vi "TestStand.Shutdown.vi"(8 "error in (no error)":errorcluster, 11 "state variables in":T1={"Main.DUTs"=[], "Pages.Name"=[], "Pages.Ref"=[], "TS.UI"={"References"={"Event Callback"=refnum, "Quit Application Event"=refnum, "Events"=refnum, "Top level VI"=refnum, "TestStand Engine"=refnum, "Start Application Event"=refnum, "Stop Application Event"=refnum}, "Managers"={"Application Manager"=refnum, "SequenceFileView Manager"=refnum, "ExecutionView Manager"=refnum}, "Controls"={"Execution View"=refnum, "Run Button"=refnum, "Open Button"=refnum}}, "TS.Running"=FALSE, "TS.Abort"=FALSE, "NIVS.GatewayIPAddress"="", "NIVS.WorkspaceManager"=refnum, "NIVS.Open"=FALSE, "NIVS.Deployed"=FALSE, "NIVS.SystemStateRefs"={"CustDatRef"=refnum, "EvtRef"=refnum, "Target State User Event"=refnum}, "NIVS.Events"={"SystemChangeEvent"=refnum, "WorkspaceEvent"=refnum, "WaveformEvent"=refnum}, "UI.Tree"=refnum, "UI.Path"=refnum, "UI.Stop"=refnum, "UI.Tab"=refnum, "VI.Ref"=refnum, "Analysis.Parameters"={"Global.ResultsPath"=path "C:/testdata/Logs", "Global.TempPath"=path "C:/testdata/Temp", "Global.RemotePath"=path "d:/testdata/Logs", "TDMS.AnalysisVIs"=[path "C:/addons/TestStand Examples for HIL/Continuous Monitoring Tester/TestStand Sequences/LabVIEW Steps/Builds/TestStand Analysis Steps.lvlibp/Post Process Analysis Steps/Analysis.LevelTransition.vi"], "TDMS.ReportPassed"=TRUE, "TDMS.GroupChannels"=TRUE}, "DUTExecution.Tabs"=[], "Overview.Columns"=[], "SharedExecution.Tabs"=[], "SharedExecution.Use"=TRUE}) -> (0 "error out":errorcluster)   [LabVIEW 2015, in "Main.GUI.lvlib"]
uses:
  Main.GUI.lvlib
  Types/Multihead.StateVariables.ctl
  Types/TestStandGUI.Refs.ctl
  <vilib>/NI Veristand/Execution/Workspace/WorkspaceAPI.ctl
  NationalInstruments.VeriStand.ClientAPI
  <vilib>/NI Veristand/Execution/Workspace/SystemStateEventRef.ctl
  <vilib>/NI Veristand/Execution/Workspace/Target State Info.ctl
  <vilib>/NI Veristand/Execution/Workspace/Target State.ctl
  Execution GUI/Types/Execute.UserEventRefs.ctl
  <vilib>/NI Veristand/Execution/Workspace/SystemStateRegEventRef.ctl
  <vilib>/NI Veristand/Execution/WaveformStreaming/Waveform Data Watcher Event Data (DBL).ctl
  <vilib>/NI Veristand/Execution/WaveformStreaming/WaveformStreamSpecification.ctl
  Analysis GUI/Types/Analysis.GUI.Parameters.ctl
  <vilib>/NI Veristand/Execution/Workspace/NI_VS Workspace ExecutionAPI.lvlib
  Execution GUI/Station.Execution.lvlib
  <vilib>/NI Veristand/Execution/WaveformStreaming/NI_VS Waveform Streaming Interface.lvlib
  Analysis GUI/Analysis.lvlib
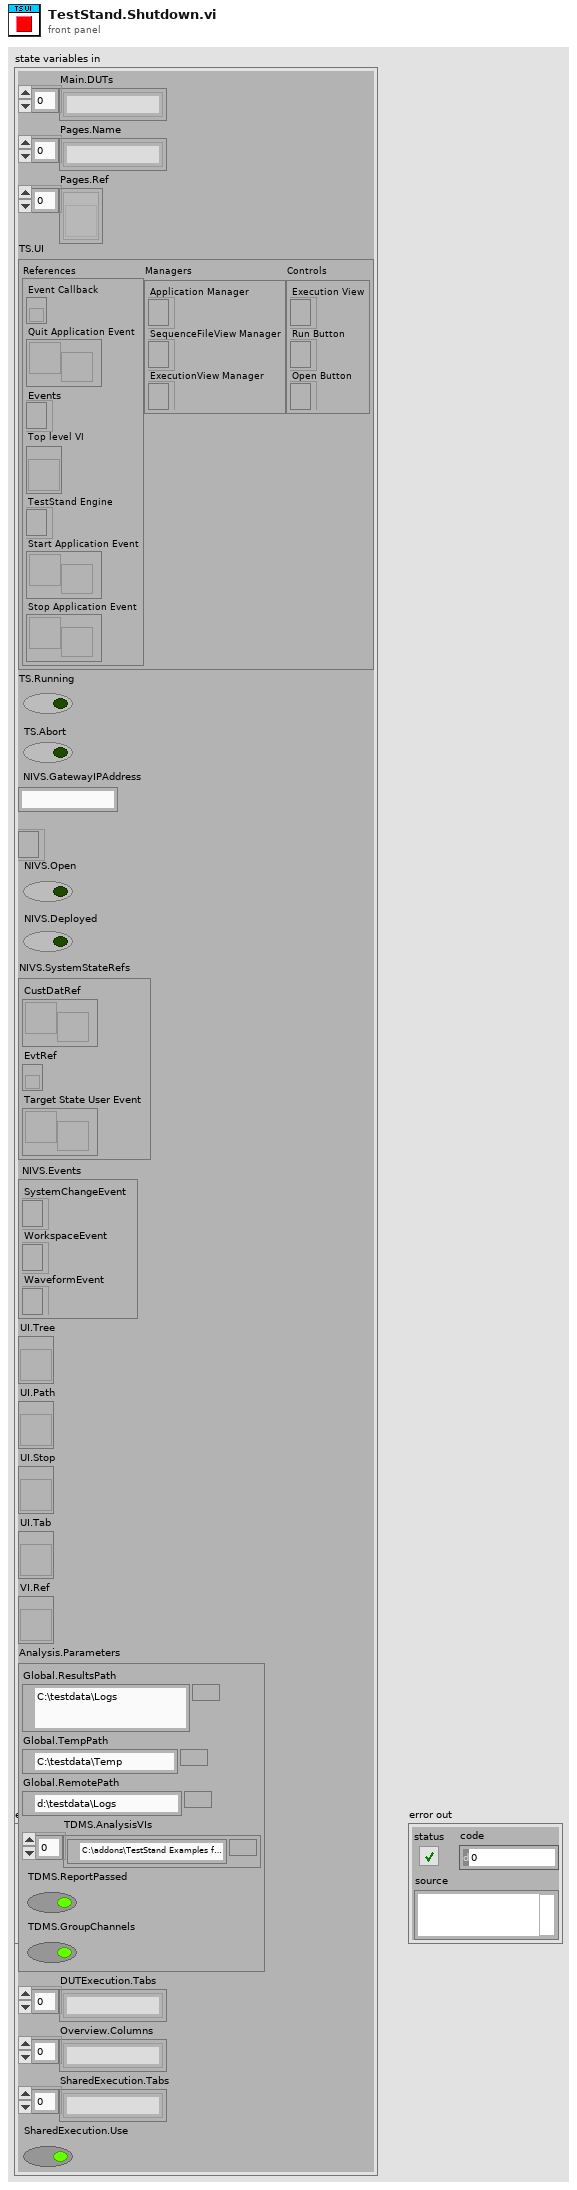
[diagram p1: front panel]
types:
  T1 = typedef "Main.GUI.lvlib/Multihead.StateVariables.ctl" = cluster{"Main.DUTs":string[], "Pages.Name":string[], "Pages.Ref":refnum<vi>[], "TS.UI":T2, "TS.Running":bool, "TS.Abort":bool, "NIVS.GatewayIPAddress":string, "NIVS.WorkspaceManager":T3, "NIVS.Open":bool, "NIVS.Deployed":bool, "NIVS.SystemStateRefs":T4, "NIVS.Events":T5, "UI.Tree":refnum<vi>, "UI.Path":refnum<vi>, "UI.Stop":refnum<vi>, "UI.Tab":refnum<vi>, "VI.Ref":refnum<vi>, "Analysis.Parameters":T7, "DUTExecution.Tabs":string[], "Overview.Columns":string[], "SharedExecution.Tabs":string[], "SharedExecution.Use":bool}
  T2 = typedef "Main.GUI.lvlib/TestStandGUI.Refs.ctl" = cluster{"References":cluster{"Event Callback":refnum<k27>, "Quit Application Event":refnum<user-event>, "Events":refnum<event-registration>, "Top level VI":refnum<vi>, "TestStand Engine":refnum<k7>, "Start Application Event":refnum<user-event>, "Stop Application Event":refnum<user-event>}, "Managers":cluster{"Application Manager":refnum<k7>, "SequenceFileView Manager":refnum<k7>, "ExecutionView Manager":refnum<k7>}, "Controls":cluster{"Execution View":refnum<k7>, "Run Button":refnum<k7>, "Open Button":refnum<k7>}}
  T3 = typedef "NI_VS Workspace ExecutionAPI.lvlib/WorkspaceAPI.ctl" = refnum<k24>
  T4 = typedef "NI_VS Workspace ExecutionAPI.lvlib/SystemStateEventRef.ctl" = cluster{"CustDatRef":refnum<user-event>, "EvtRef":refnum<k27>, "Target State User Event":refnum<user-event>}
  T5 = typedef "Station.Execution.lvlib/Execute.UserEventRefs.ctl" = cluster{"SystemChangeEvent":T6, "WorkspaceEvent":refnum<event-registration>, "WaveformEvent":refnum<event-registration>}
  T6 = typedef "NI_VS Workspace ExecutionAPI.lvlib/SystemStateRegEventRef.ctl" = refnum<event-registration>
  T7 = typedef "Analysis.lvlib/Analysis.GUI.Parameters.ctl" = cluster{"Global.ResultsPath":path, "Global.TempPath":path, "Global.RemotePath":path, "TDMS.AnalysisVIs":path[], "TDMS.ReportPassed":bool, "TDMS.GroupChannels":bool}
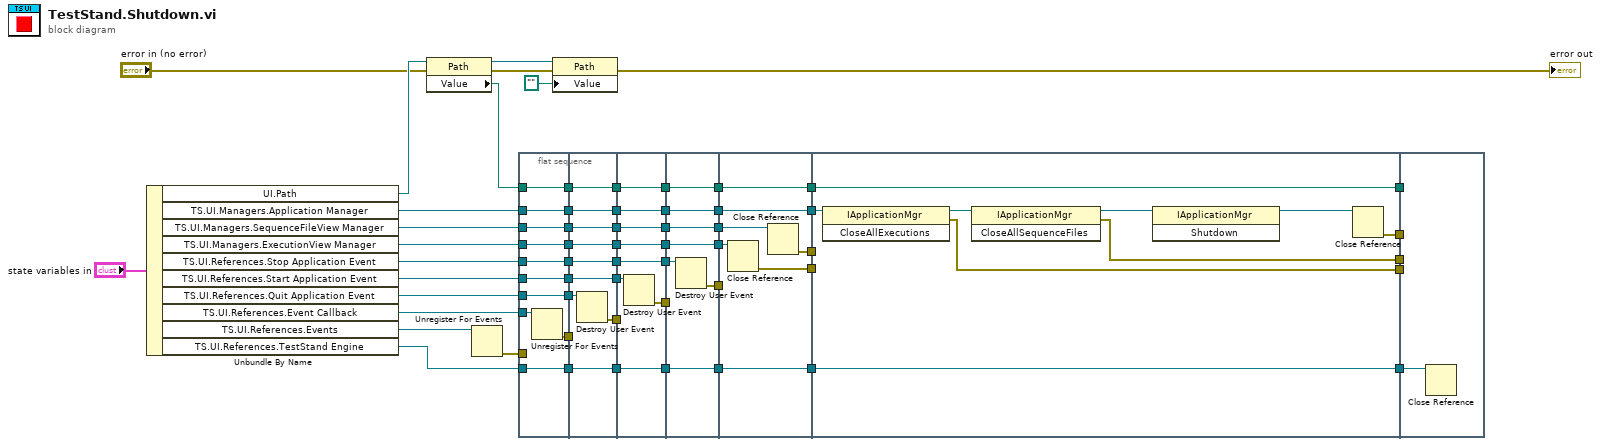
[diagram p0: block diagram]
diagram:
  n1 = Unbundle By Name("state variables in") -> ("UI.Path"=w19:refnum<vi>, "TS.UI.Managers.Application Manager"=w20:refnum<k7>, "TS.UI.Managers.SequenceFileView Manager"=w21:refnum<k7>, "TS.UI.Managers.ExecutionView Manager"=w22:refnum<k7>, "TS.UI.References.Stop Application Event"=w23:refnum<user-event>, "TS.UI.References.Start Application Event"=w17:refnum<user-event>, "TS.UI.References.Quit Application Event"=w14:refnum<user-event>, "TS.UI.References.Event Callback"=w12:refnum<k27>, "TS.UI.References.Events"=w13:refnum<event-registration>, "TS.UI.References.TestStand Engine"=w24:refnum<k7>)
  n2 = property class="Path"(reference=w19, error in="error in (no error)") -> (reference out=w2:refnum<vi>, error out=w4:errorcluster, "Value"=w11:path)
  n3 = Unregister For Events(event registration refnum=w13) -> (error out=w15:errorcluster)  [unwired: 1 in]
  n4 = flat-sequence {
    tunnel: w12 -> [w68]
    tunnel: [w67] -> w58
    tunnel: w14 -> [w67]
    tunnel: w15 -> [_]
    tunnel: [w66] -> w57
    tunnel: [w65] -> w56
    tunnel: w17 -> [w65]
    tunnel: [w64] -> w55
    tunnel: w20 -> [w64]
    tunnel: [w63] -> w54
    tunnel: w21 -> [w63]
    tunnel: [w62] -> w53
    tunnel: w22 -> [w62]
    tunnel: [w61] -> w52
    tunnel: w23 -> [w61]
    tunnel: [w60] -> w51
    tunnel: w24 -> [w60]
    tunnel: w11 -> [w59]
    tunnel: [w59] -> w5
    tunnel: w58 -> [w77]
    tunnel: w57 -> [_]
    tunnel: [w76] -> w50
    tunnel: [w75] -> w49
    tunnel: w56 -> [w75]
    tunnel: [w74] -> w48
    tunnel: w55 -> [w74]
    tunnel: [w73] -> w47
    tunnel: w54 -> [w73]
    tunnel: [w72] -> w46
    tunnel: w53 -> [w72]
    tunnel: [w71] -> w45
    tunnel: w52 -> [w71]
    tunnel: [w70] -> w44
    tunnel: w51 -> [w70]
    tunnel: [w69] -> w6
    tunnel: w5 -> [w69]
    tunnel: w50 -> [_]
    tunnel: w49 -> [w85]
    tunnel: [w84] -> w43
    tunnel: [w83] -> w42
    tunnel: w48 -> [w83]
    tunnel: [w82] -> w41
    tunnel: w47 -> [w82]
    tunnel: [w81] -> w40
    tunnel: w46 -> [w81]
    tunnel: [w80] -> w39
    tunnel: w45 -> [w80]
    tunnel: [w79] -> w38
    tunnel: w44 -> [w79]
    tunnel: [w78] -> w7
    tunnel: w6 -> [w78]
    tunnel: w43 -> [_]
    tunnel: w42 -> [w92]
    tunnel: [w92] -> w37
    tunnel: w41 -> [w91]
    tunnel: [w91] -> w36
    tunnel: w40 -> [w90]
    tunnel: [w90] -> w35
    tunnel: w39 -> [w89]
    tunnel: [w88] -> w34
    tunnel: [w87] -> w33
    tunnel: w38 -> [w87]
    tunnel: [w86] -> w8
    tunnel: w7 -> [w86]
    tunnel: w37 -> [w95]
    tunnel: w36 -> [w99]
    tunnel: w35 -> [w98]
    tunnel: w34 -> [_]
    tunnel: [w97] -> w32
    tunnel: [w96] -> w31
    tunnel: [w95] -> w30
    tunnel: [w94] -> w29
    tunnel: w33 -> [w94]
    tunnel: [w93] -> w9
    tunnel: w8 -> [w93]
    tunnel: w32 -> [_]
    tunnel: w31 -> [_]
    tunnel: w30 -> [w104]
    tunnel: [w107] -> w28
    tunnel: [w106] -> w27
    tunnel: [w105] -> w26
    tunnel: [w103] -> w25
    tunnel: w29 -> [w103]
    tunnel: [w102] -> w10
    tunnel: w9 -> [w102]
    tunnel: w28 -> [_]
    tunnel: w27 -> [_]
    tunnel: w26 -> [_]
    tunnel: w25 -> [w109]
    tunnel: w10 -> [_]
    frame #0 {
      n5 = Unregister For Events(event registration refnum=w68) -> (error out=w66:errorcluster)  [unwired: 1 in]
    }
    frame #1 {
      n6 = Destroy User Event(user event=w77) -> (error out=w76:errorcluster)  [unwired: 1 in]
    }
    frame #2 {
      n7 = Destroy User Event(user event=w85) -> (error out=w84:errorcluster)  [unwired: 1 in]
    }
    frame #3 {
      n8 = Destroy User Event(user event=w89) -> (error out=w88:errorcluster)  [unwired: 1 in]
    }
    frame #4 {
      n9 = Close Reference(reference=w98) -> (error out=w97:errorcluster)  [unwired: 1 in]
      n10 = Close Reference(reference=w99) -> (error out=w96:errorcluster)  [unwired: 1 in]
    }
    frame #5 {
      n11 = invoke class="IApplicationMgr" method="CloseAllExecutions"(reference=w104) -> (reference out=w108:refnum<k7>, error out=w107:errorcluster)  [unwired: 2 in, 1 out]
      n12 = invoke class="IApplicationMgr" method="CloseAllSequenceFiles"(reference=w108) -> (reference out=w101:refnum<k7>, error out=w106:errorcluster)  [unwired: 2 in, 1 out]
      n13 = invoke class="IApplicationMgr" method="Shutdown"(reference=w101) -> (reference out=w100:refnum<k7>)  [unwired: 2 in, 2 out]
      n14 = Close Reference(reference=w100) -> (error out=w105:errorcluster)  [unwired: 1 in]
    }
    frame #6 {
      n15 = Close Reference(reference=w109) -> ()  [unwired: 1 in, 1 out]
    }
  }
  n16 = property class="Path"(reference=w2, error in=w4, "Value"=path "") -> (error out=→"error out":errorcluster)  [unwired: 1 out]
